vi "Try to Take a Measurement.vi"(0 "Register Buses":T1[](array[typedef]), 1 "Max Attempts":u32=10, 11 "error in":errorcluster) -> (4 "Register Buses (out)":T1[](array[typedef]), 6 "measurement values":u16[](array[numeric]), 15 "error out":errorcluster)   [LabVIEW 2014, in "ni579x Synchronization v2 Host.lvlib"]
uses:
  <instrlib>/ni579x/Synchronization/v2/Host/ni579x Synchronization v2 Host.lvlib
  <instrlib>/_niInstr/Register Bus/v0/Host/Public/Register Bus Session.ctl
  <instrlib>/_niInstr/Register Bus/v0/Host/Private/Session Data.ctl
  <vilib>/ErrorRing/Error Ring.xnode
  <instrlib>/_niInstr/Register Bus/v0/Host/niInstr Register Bus v0 Host.lvlib
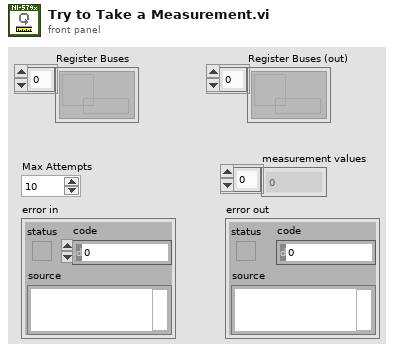
[diagram p1: front panel]
types:
  T1 = typedef "niInstr Register Bus v0 Host.lvlib/Register Bus Session.ctl" = refnum<queue>
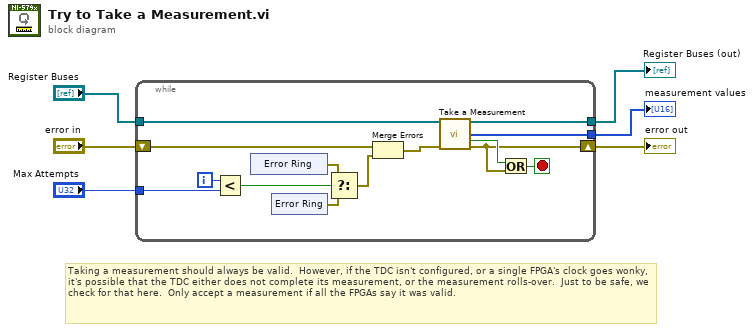
[diagram p0: block diagram]
diagram:
  # "Taking a measurement should always be valid.  However, if the TDC isn't configured, or a single FPGA's clock goes wonky, it's possible that the TDC either does not complete its measurement, or the measurement rolls-over.  Just to be safe, we check for that here.  Only accept a measurement if all the FPGAs say it was valid."
  n1 = while {
    tunnel: [w9] -> w6
    tunnel: "Max Attempts" -> [w17]
    tunnel: "Register Buses" -> [w8]
    tunnel: [w7] -> w1
    shift-right: [w18] -> w5
    shift-left: "error in" -> [w11]
    i -> [w16]
    stop <- w20 stop-if-true
    n2 = Less?(x=w16, y=w17) -> (x < y?=w10:bool)
    n3 = xnode ("Error Ring")() -> ("error out"=w14:errorcluster)
    n4 = xnode ("Error Ring")() -> ("error out"=w15:errorcluster)
    n5 = Select(t=w14, s=w10, f=w15) -> (s? t:f=w13:errorcluster)
    n6 = Merge Errors(w11, w13) -> (w12:errorcluster)
    n7 = call <instrlib>:"Take a Measurement.vi"("Register Buses"=w8, "error in"=w12) -> ("Register Buses (out)"=w7:T1[], "measurement values"=w9:u16[], "measurement valid"=w19:bool, "error out"=w18:errorcluster)  [unwired: 10 in]
    n8 = Or(x=w19, y=w18) -> (x .or. y?=w20:bool)
  }
  "measurement values" <- w6
  "error out" <- w5
  "Register Buses (out)" <- w1
